vi "ex_3b.vi"() -> ()   [LabVIEW 2020]
uses:
  <vilib>/numeric/Random Number (Range) U64.vi
  <vilib>/numeric/sub_Random U32.vi
panel:
  out "Result 2":u64[](array[numeric])
  out "Array K":u64[](array[numeric])
  out "Array M":u64[](array[numeric])
  in  "K":i32
  in  "M":i32
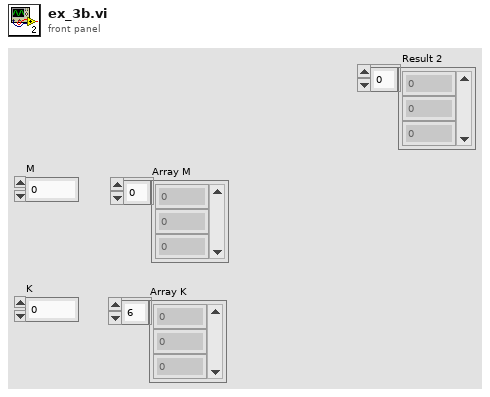
[diagram p1: front panel]
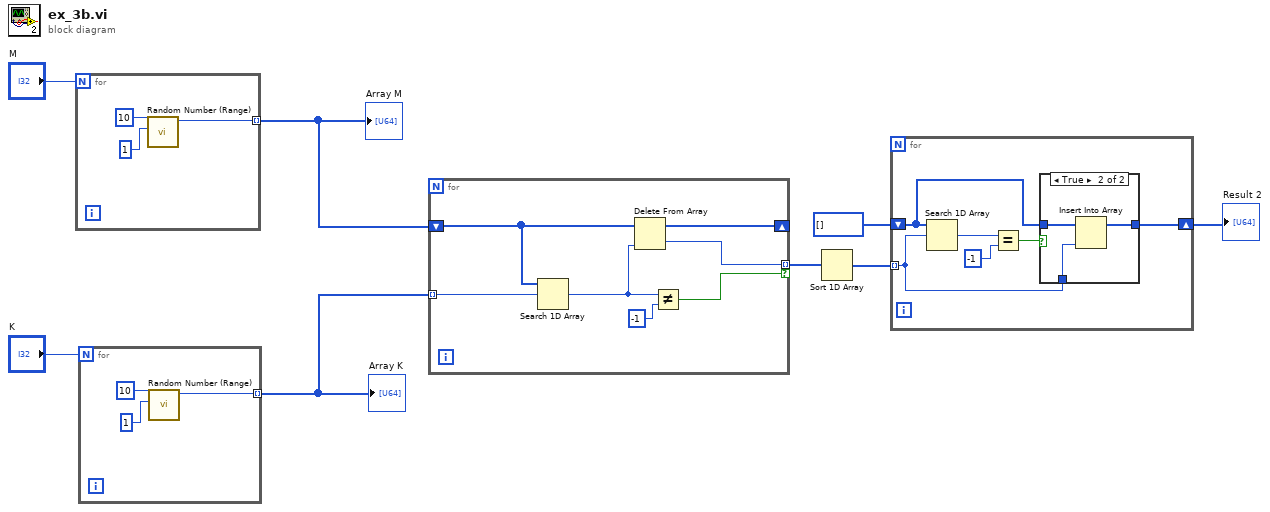
[diagram p0: block diagram]
diagram:
  n1 = for {
    N: "M" -> [_]
    tunnel: [w9] -> w5 mode=indexing
    n2 = call-poly <vilib>:"Random Number (Range).vi"("lower bound (0)"=u64 1, "upper bound (100)"=u64 10) -> ("number"=w9:u64)  [unwired: 9 in]
  }
  "Array M" <- w5
  n3 = for {
    N: "K" -> [_]
    tunnel: [w12] -> w6 mode=indexing
    n4 = call-poly <vilib>:"Random Number (Range).vi"("lower bound (0)"=u64 1, "upper bound (100)"=u64 10) -> ("number"=w12:u64)  [unwired: 9 in]
  }
  "Array K" <- w6
  n5 = for {
    tunnel: w6 -> [w21] mode=indexing
    shift-right: [w19] -> _
    shift-left: w5 -> [w20]
    tunnel: [w16] -> w4 mode=indexing if=w15
    n6 = Search 1D Array(1D array=w20, element=w21) -> (index of element=w18:i32)  [unwired: 1 in]
    n7 = Delete From Array(array=w20, index=w18) -> (deleted portion=w16:u64, array with subset deleted=w19:u64[])  [unwired: 1 in]
    n8 = Not Equal?(x=w18, y=-1) -> (x != y?=w15:bool)
  }
  n9 = Sort 1D Array(array=w4) -> (sorted array=w3:u64[])
  n10 = for {
    tunnel: w3 -> [w22] mode=indexing
    shift-right: [w24] -> w1
    shift-left: u64[] [] ("Result 2") -> [w23]
    n11 = Search 1D Array(1D array=w23, element=w22) -> (index of element=w26:i32)  [unwired: 1 in]
    n12 = Equal?(x=w26, y=-1) -> (x = y?=w25:bool)
    n13 = case shown="True" w25 {
      tunnel: [w28 w30] -> w24
      tunnel: w23 -> [w28 w31]
      tunnel: w22 -> [_ w29]
      frame False {
      }
      frame True {
        n14 = Insert Into Array(array=w31, new element=w29) -> (w30:u64[])  [unwired: 1 in]
      }
    }
  }
  "Result 2" <- w1
